vi "Global Coppia letta.vi"() -> ()   [LabVIEW 2019]
panel:
  out "C [NM] simulata":dbl
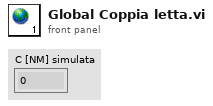
[diagram p1: front panel]
diagram:
